vi "HandeSignals.vi"(0 "reference in":refnum<class "Logger.lvclass">, 11 "error in (no error)":errorcluster) -> (4 "reference out":refnum<class "Logger.lvclass">, 14 "dt":u32, 15 "error out":errorcluster)   [LabVIEW 2019, in "Logger.lvclass"]
uses:
  Logger.lvclass
  SignalData.ctl
  TypeDef/engineering units.ctl
  Logger.lvclass/Logger.ctl
  2f3f98d4-cfb0-4f81-b92a-0d178dd61f1e.vi
  1c0d0c3d-5d6b-42fa-8895-123650284108.vi
  DatabaseInterface_class/DatabaseInterface.lvclass
panel:
  out "remaining elements":T1[](array[typedef])
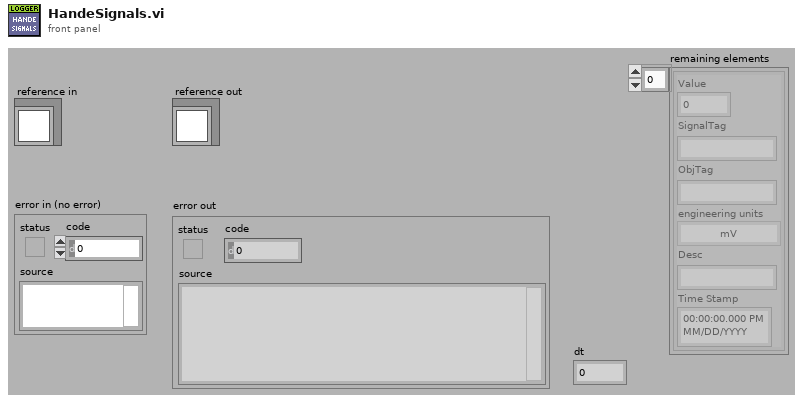
[diagram p1: front panel]
types:
  T1 = typedef "Logger.lvclass/SignalData.ctl" = cluster{"Value":dbl, "SignalTag":string, "ObjTag":string, "engineering units":T2, "Desc":string, "Time Stamp":timestamp}
  T2 = typedef "engineering units.ctl" = enum16{"mV", "V", "mA", "A", "C", "pC", "s", "Pa", "N", "g", "m/s^2", "m/s", "m", "mm/s", "mm", "micron/s", "micron", "in/s^2", "in/s", "in", "mil/s", "mil", "rad/s^2", "rad/s", "rad", "deg/s^2", "deg/s", "deg", "RPM", "cycle/s^2", "Hz", "cycle", "strain", "%"}
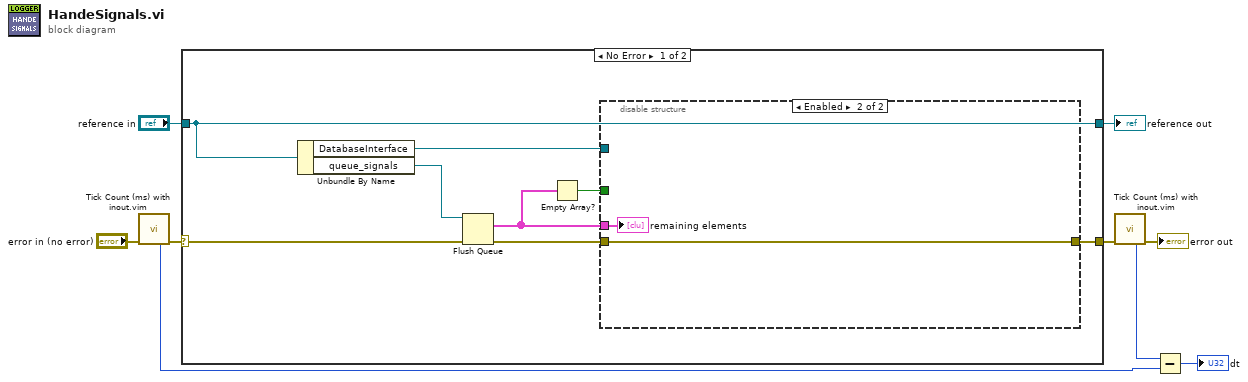
[diagram p0: block diagram]
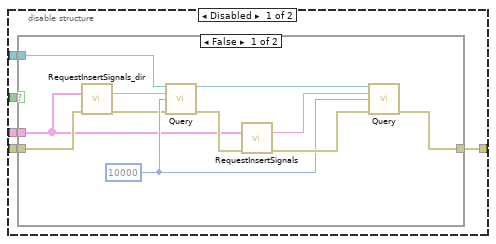
[diagram p2: hidden frame]
diagram:
  n1 = call "Tick Count (ms) with inout.vim"("in"="error in (no error)") -> ("millisecond timer value dub"=w4:u32, "out"=w7:errorcluster)  [unwired: 12 in, 1 out]
  n2 = case shown="No Error" w7 {
    selector: w7 -> [w17 w37]
    tunnel: [w16 w38] -> w2
    tunnel: "reference in" -> [w16 w38]
    tunnel: [w14 w37] -> w1
    frame No Error {
      n3 = Unbundle By Name(w16) -> ("DatabaseInterface"=w12:refnum<class "DatabaseInterface.lvclass">, "queue_signals"=w15:refnum<queue>)
      n4 = Flush Queue(queue=w15, error in (no error)=w17) -> (remaining elements=w11:T1[], error out=w13:errorcluster)  [unwired: 1 out]
      n5 = Empty Array?(array=w11) -> (empty?=w10:bool)
      n6 = disable-structure shown="Enabled" {
        disable-tunnel: [w22 w36] -> w14
        disable-tunnel: w13 -> [w21 w36]
        disable-tunnel: w12 -> [w20 _]
        disable-tunnel: w11 -> [w19 w35]
        disable-tunnel: w10 -> [w18 _]
        frame Disabled {
          n7 = case shown="False" w18 {
            tunnel: [w33 w34] -> w22
            tunnel: w21 -> [w32 w34]
            tunnel: w20 -> [w27 _]
            tunnel: w19 -> [w23 _]
            frame False {
              w28 = 10000 ("Timeout")
              n8 = call "RequestInsertSignals_dir.vi"("Events"=w23, "error in (no error)"=w32) -> ("request"=w29:string, "error out"=w25:errorcluster)  [unwired: 12 in]
              n9 = call-dynamic "Query.vi"("reference in"=w27, "Query"=w29, "Timeout"=w28, "error in (no error)"=w25) -> ("reference out"=w26:refnum<class "DatabaseInterface.lvclass">, "error out"=w24:errorcluster)  [unwired: 9 in, 1 out]
              n10 = call "RequestInsertSignals.vi"("Events"=w23, "error in (no error)"=w24) -> ("request"=w30:string, "error out"=w31:errorcluster)  [unwired: 12 in]
              n11 = call-dynamic "Query.vi"("reference in"=w26, "Query"=w30, "Timeout"=w28, "error in (no error)"=w31) -> ("error out"=w33:errorcluster)  [unwired: 9 in, 2 out]
            }
            frame True {
            }
          }
        }
        frame Enabled {
          "remaining elements" <- w35
        }
      }
    }
    frame Error {
    }
  }
  "reference out" <- w2
  n12 = call "Tick Count (ms) with inout.vim"("in"=w1) -> ("millisecond timer value dub"=w5:u32, "out"=→"error out":errorcluster)  [unwired: 12 in, 1 out]
  n13 = Subtract(x=w5, y=w4) -> (x-y=→"dt":u32)
